vi "Insert.vi"() -> ()   [LabVIEW 2013]
doc: "This VI show interleaver of array."
panel:
  out "interleaved array":i32[](array[numeric])
  out "b":i32[](array[numeric])
  out "a":i32[](array[numeric])
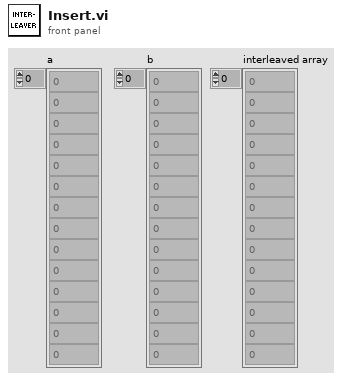
[diagram p1: front panel]
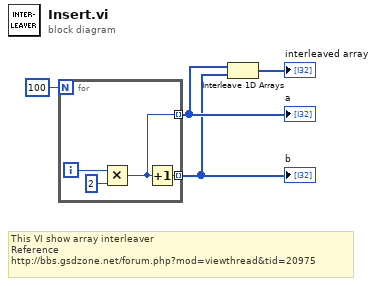
[diagram p0: block diagram]
diagram:
  # "This VI show array interleaver\nReference\nhttp://bbs.gsdzone.net/forum.php?mod=viewthread&tid=20975"
  n1 = for {
    N: 100 -> [_]
    tunnel: [w6] -> w1 mode=indexing
    tunnel: [w5] -> w2 mode=indexing
    i -> [w7]
    n2 = Multiply(x=w7, y=2) -> (x*y=w5:i32)
    n3 = Increment(x=w5) -> (x+1=w6:i32)
  }
  "a" <- w2
  "b" <- w1
  n4 = Interleave 1D Arrays(w2, w1) -> (→"interleaved array":i32[])
